vi "ZstageConnectTest.vi"() -> ()   [LabVIEW 2018]
uses:
  C:/Project/SerialSectOCT - FFT GPU/SerialSectOCT/Labview Software/Thorlabs.MotionControl.Controls.dll
  Thorlabs.MotionControl.Controls.dll
  Hardware Mfg/Thorlabs Translation Stages/Controls/Translation Stage Cluster.ctl
  General/Controls/Translation Stage Types.ctl
panel:
  out "IsConnected":bool
  in  "Cluster in 2":T1
  in  "error in (no error)":errorcluster
  out "MLJ Reference Out":refnum<k24>
  out "Cluster out":T1
  out "error out":errorcluster
  in  "LabJackControl":refnum<k24>(container)
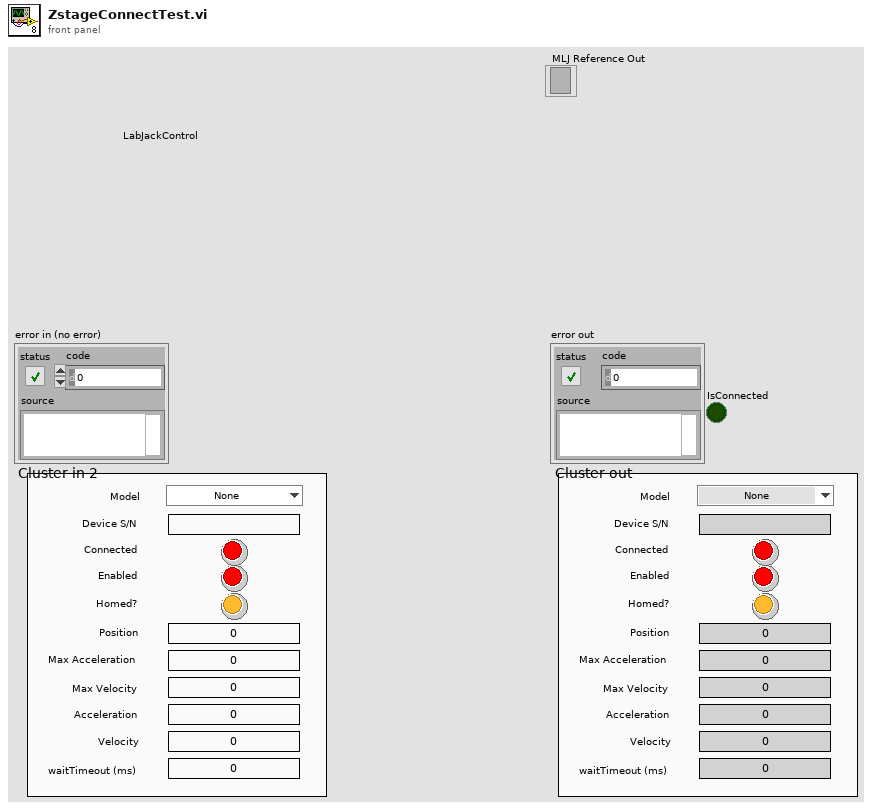
[diagram p1: front panel]
types:
  T1 = typedef "Translation Stage Cluster.ctl" = cluster{"Position":dbl, "Is.Enabled?":bool, "Is.Connected?":bool, "Device SN":string, "AccelerationMaximum":dbl, "VelocityMaximum":dbl, "Acceleration":dbl, "Velocity":dbl, "waitTimeout (ms)":i32, "Model":T2, "Is.Homed?":bool}
  T2 = typedef "Translation Stage Types.ctl" = enum16{"None", "Thorlabs LTS", "Thorlabs MLJ"}
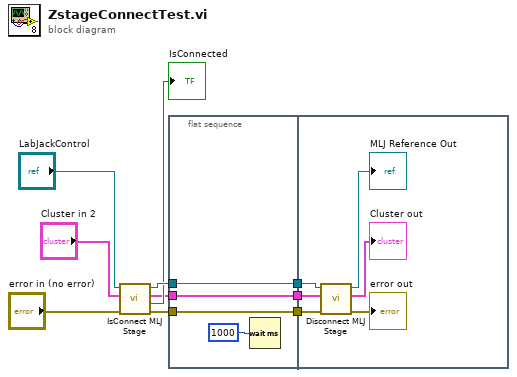
[diagram p0: block diagram]
diagram:
  n1 = call "IsConnect MLJ Stage.vi"("error in (no error)"="error in (no error)", "Cluster in"="Cluster in 2", "MLJ Reference In"="LabJackControl") -> ("error out"=w8:errorcluster, "IsConnected"=→"IsConnected":bool, "Cluster out"=w1:T1, "MLJ Reference Out"=w9:refnum<k24>)  [unwired: 5 in]
  n2 = flat-sequence {
    tunnel: w8 -> [w13]
    tunnel: w9 -> [w14]
    tunnel: [w14] -> w7
    tunnel: [w13] -> w6
    tunnel: [w11] -> w2
    tunnel: w1 -> [w11]
    tunnel: w7 -> [w20]
    tunnel: w6 -> [w19]
    tunnel: w2 -> [w15]
    frame #0 {
      n3 = Wait (ms)(milliseconds to wait=u32 1000) -> ()  [unwired: 1 out]
    }
    frame #1 {
      n4 = call "Disconnect MLJ Stage.vi"("error in (no error)"=w19, "Cluster in"=w15, "MLJ Reference In"=w20) -> ("error out"=→"error out":errorcluster, "Cluster out"=→"Cluster out":T1, "MLJ Reference Out"=→"MLJ Reference Out":refnum<k24>)  [unwired: 6 in]
    }
  }
